vi "test Validate Existing Connections.vi"(8 "error in (no error)":errorcluster, 11 "TestCase in":refnum<class "Routing and Faulting Validation Unit Tests.lvclass">) -> (0 "error out":errorcluster, 3 "TestCase out":refnum<class "Routing and Faulting Validation Unit Tests.lvclass">)   [LabVIEW 2020, in "Routing and Faulting Validation Unit Tests.lvclass"]
uses:
  Routing and Faulting Validation Unit Tests.lvclass
  Routing and Faulting Validation Unit Tests.lvclass/Routing and Faulting Validation Unit Tests.ctl
  <vilib>/addons/_JKI Toolkits/VI Tester/TestCase.llb/TestCase.lvclass
  Routing and Faulting Scripting.lvlib
  C:/Program Files (x86)/National Instruments/LabVIEW 2020/vi.lib/addons/_JKI Toolkits/VI Tester/TestCase.llb/TestCase.lvclass
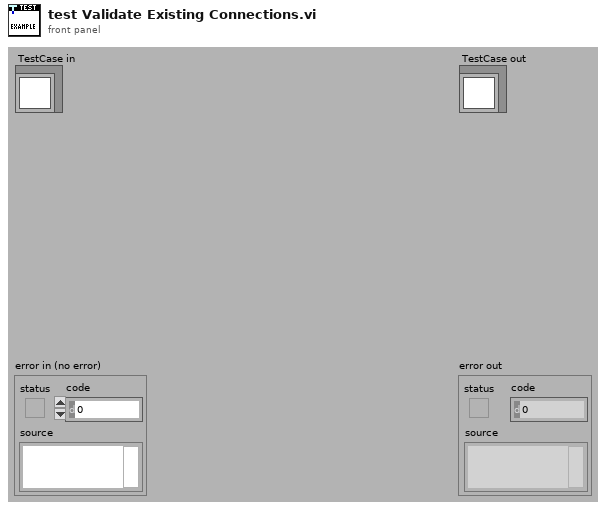
[diagram p1: front panel]
types:
  T1 = cluster{"channel":string, "state":string, "resource":string}[]
  T2 = typedef "Custom Device API.lvlib/Custom Device Item Ref.ctl" = u64
  T3 = typedef "Routing and Faulting Scripting.lvlib/Validation Information.ctl" = cluster{"Missing Modules":variant, "Module Connection Map":variant, "Unused Modules":variant}
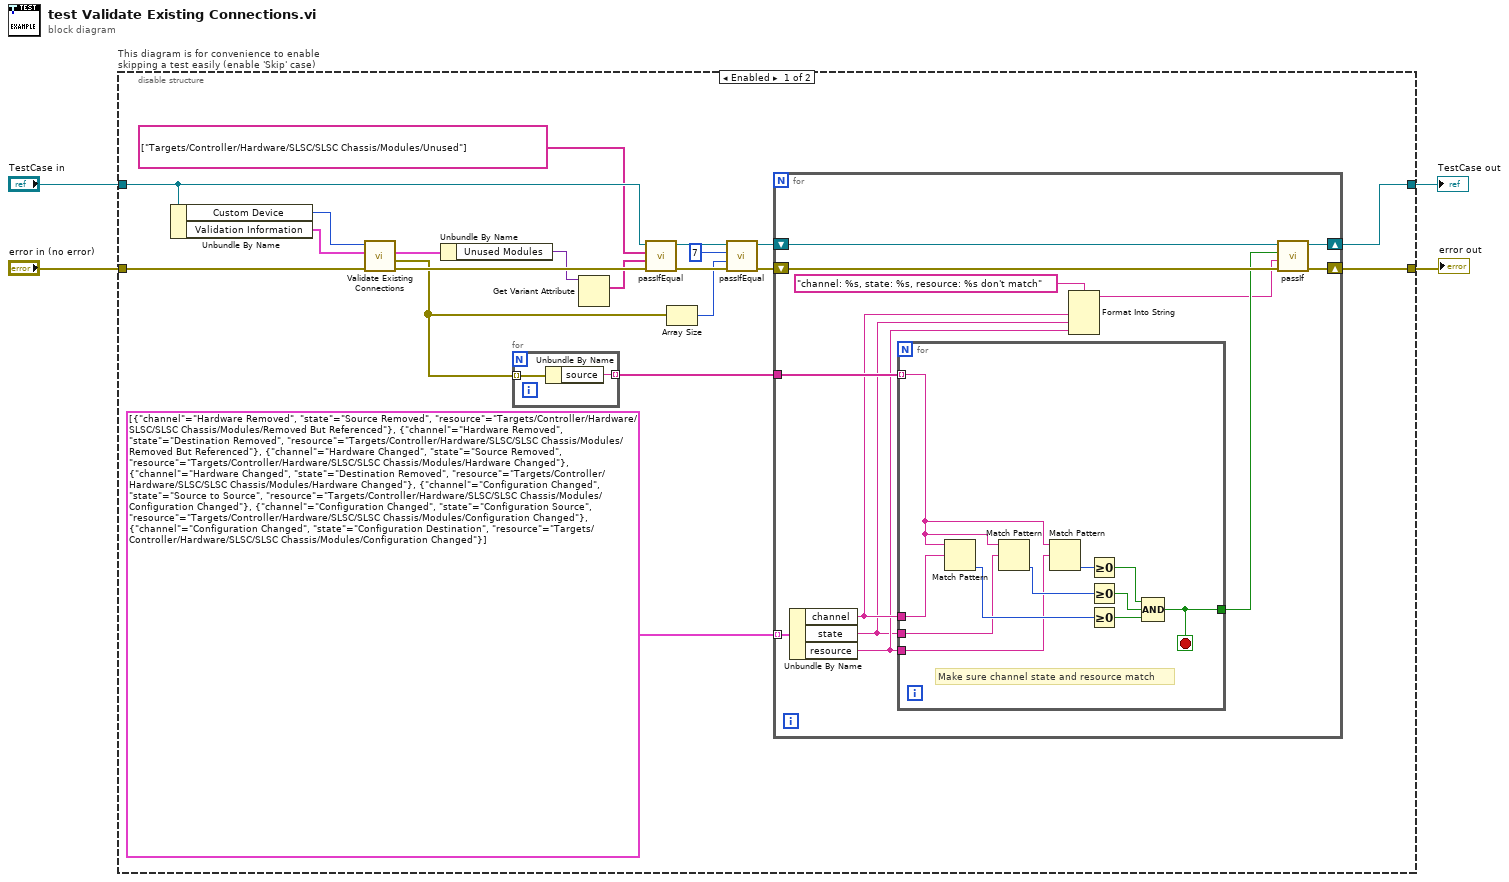
[diagram p0: block diagram]
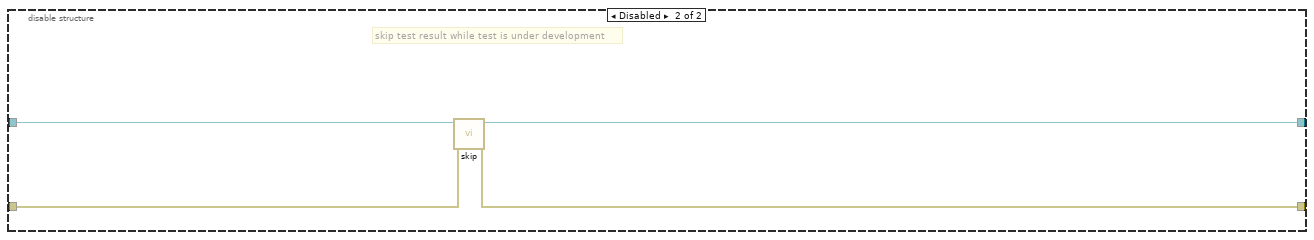
[diagram p2: hidden frame]
diagram:
  n1 = disable-structure "This diagram is for convenience to enable skipping a test easily (enable 'Skip' case)" shown="Enabled" {
    disable-tunnel: "TestCase in" -> [w17 w53]
    disable-tunnel: [w5 w51] -> w1
    disable-tunnel: [w6 w52] -> w3
    disable-tunnel: "error in (no error)" -> [w24 w50]
    frame Enabled {
      n2 = Unbundle By Name(w17) -> ("Custom Device"=w21:T2, "Validation Information"=w22:T3)
      n3 = call "Validate Existing Connections.vi"("error in"=w24, "validation information in"=w22, "routing and faulting in"=w21) -> ("error out"=w23:errorcluster, "connection errors"=w11:errorcluster[], "validation information out"=w20:T3)  [unwired: 5 in, 1 out]
      n4 = Unbundle By Name(w20) -> ("Unused Modules"=w19:variant)
      n5 = for {
        tunnel: w11 -> [w49] mode=indexing
        tunnel: [w48] -> w8 mode=indexing
        n6 = Unbundle By Name(w49) -> ("source"=w48:string)
      }
      n7 = Get Variant Attribute(Variant=w19) -> (names=w15:string[])  [unwired: 3 in, 3 out]
      n8 = call-dynamic "passIfEqual.vi"("error in (no error)"=w23, "y"=w15, "x"=string[] ["Targets/Controller/Hardware/SLSC/SLSC Chassis/Modules/Unused"] ("names"), "TestCase in"=w17) -> ("error out"=w18:errorcluster, "TestCase out"=w13:refnum<class "Routing and Faulting Validation Unit Tests.lvclass">)  [unwired: 6 in]
      n9 = Array Size(array=w11) -> (size(s)=w14:i32)
      n10 = call-dynamic "passIfEqual.vi"("error in (no error)"=w18, "y"=w14, "x"=7 ("size(s)"), "TestCase in"=w13) -> ("error out"=w10:errorcluster, "TestCase out"=w9:refnum<class "Routing and Faulting Validation Unit Tests.lvclass">)  [unwired: 6 in]
      n11 = for {
        shift-right: [w33] -> w6
        shift-left: w10 -> [w34]
        shift-right: [w30] -> w5
        shift-left: w9 -> [w31]
        tunnel: w8 -> [w36]
        tunnel: T1 [{"channel"="Hardware Removed", "state"="Source Removed", "resource"="Targets/Controller/Hardware/SLSC/SLSC Chassis/Modules/Removed But Referenced"}, {"channel"="Hardware Removed", "state"="Destination Removed", "resource"="Targets/Controller/Hardware/SLSC/SLSC Chassis/Modules/Removed But Referenced"}, {"channel"="Hardware Changed", "state"="Source Removed", "resource"="Targets/Controller/Hardware/SLSC/SLSC Chassis/Modules/Hardware Changed"}, {"channel"="Hardware Changed", "state"="Destination Removed", "resource"="Targets/Controller/Hardware/SLSC/SLSC Chassis/Modules/Hardware Changed"}, {"channel"="Configuration Changed", "state"="Source to Source", "resource"="Targets/Controller/Hardware/SLSC/SLSC Chassis/Modules/Configuration Changed"}, {"channel"="Configuration Changed", "state"="Configuration Source", "resource"="Targets/Controller/Hardware/SLSC/SLSC Chassis/Modules/Configuration Changed"}, {"channel"="Configuration Changed", "state"="Configuration Destination", "resource"="Targets/Controller/Hardware/SLSC/SLSC Chassis/Modules/Configuration Changed"}] -> [w35] mode=indexing
        n12 = Unbundle By Name(w35) -> ("channel"=w28:string, "state"=w26:string, "resource"=w27:string)
        n13 = for {
          tunnel: w36 -> [w39] mode=indexing
          tunnel: w28 -> [w43]
          tunnel: w26 -> [w42]
          tunnel: w27 -> [w38]
          tunnel: [w37] -> w32
          stop <- w37 stop-if-true
          # "Make sure channel state and resource match"
          n14 = Match Pattern(string=w39, regular expression=w43) -> (offset past match=w47:i32)  [unwired: 1 in, 3 out]
          n15 = Match Pattern(string=w39, regular expression=w42) -> (offset past match=w46:i32)  [unwired: 1 in, 3 out]
          n16 = Match Pattern(string=w39, regular expression=w38) -> (offset past match=w41:i32)  [unwired: 1 in, 3 out]
          n17 = Greater Or Equal To 0?(x=w41) -> (x >= 0?=w40:bool)
          n18 = Greater Or Equal To 0?(x=w46) -> (x >= 0?=w45:bool)
          n19 = Greater Or Equal To 0?(x=w47) -> (x >= 0?=w44:bool)
          n20 = Compound Arithmetic op=AND(w40, w45, w44) -> (w37:bool)
        }
        n21 = Format Into String(format string="channel: %s, state: %s, resource: %s don't match", w28, w26, w27) -> (resulting string=w25:string)  [unwired: 2 in, 1 out]
        n22 = call-dynamic "passIf.vi"("error in (no error)"=w34, "message (\"\")"=w25, "pass"=w32, "TestCase in"=w31) -> ("error out"=w33:errorcluster, "TestCase out"=w30:refnum<class "Routing and Faulting Validation Unit Tests.lvclass">)  [unwired: 6 in]
      }
    }
    frame Disabled {
      # "skip test result while test is under development"
      n23 = call <vilib>:"skip.vi"("error in (no error)"=w50, "TestCase in"=w53) -> ("error out"=w52:errorcluster, "TestCase out"=w51:refnum<class "Routing and Faulting Validation Unit Tests.lvclass">)  [unwired: 8 in]
    }
  }
  "error out" <- w3
  "TestCase out" <- w1
